vi "Show UI If Necessary.vi"(8 "error in (no error)":errorcluster, 11 "Output Sequencer in":refnum<class "Output Sequencer.lvclass">) -> (0 "error out":errorcluster, 3 "Output Sequencer out":refnum<class "Output Sequencer.lvclass">)   [LabVIEW 2024, in "Output Sequencer.lvlib" / "Output Sequencer.lvclass"]
uses:
  Output Sequencer.lvclass
  Output Sequencer.lvclass/Output Sequencer.ctl
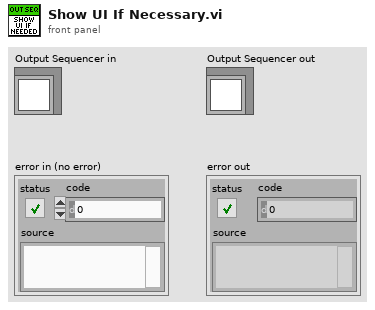
[diagram p1: front panel]
types:
  T1 = typedef "Output Sequencer.lvlib/Output Sequencer.lvclass/UI Ref.ctl" = refnum<vi>
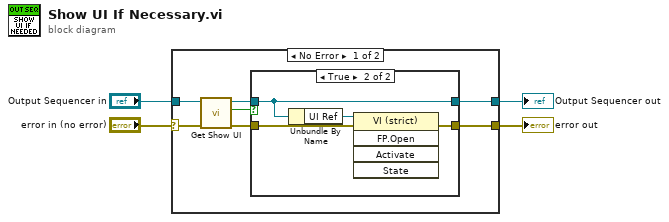
[diagram p0: block diagram]
diagram:
  n1 = case shown="No Error" "error in (no error)" {
    selector: "error in (no error)" -> [w5 w19]
    tunnel: [w11 w19] -> w4
    tunnel: [w10 w18] -> w3
    tunnel: "Output Sequencer in" -> [w6 w18]
    frame No Error {
      n2 = call "Get Show UI.vi"("error in (no error)"=w5, "Output Sequencer in"=w6) -> ("error out"=w9:errorcluster, "Show UI"=w7:bool, "Output Sequencer out"=w8:refnum<class "Output Sequencer.lvclass">)  [unwired: 7 in]
      n3 = case shown="True" w7 {
        tunnel: w8 -> [w13 w16]
        tunnel: [w13 w16] -> w10
        tunnel: w9 -> [w12 w15]
        tunnel: [w12 w14] -> w11
        frame False {
        }
        frame True {
          n4 = Unbundle By Name(w16) -> ("UI Ref"=w17:T1)
          n5 = invoke class="VI (strict)" method="FP.Open"(reference=w17, error in=w15) -> (error out=w14:errorcluster)  [unwired: 3 in, 4 out]
        }
      }
    }
    frame Error {
    }
  }
  "error out" <- w4
  "Output Sequencer out" <- w3
